vi "GetFltrMode.vi"(8 "错误输入（无错误）":errorcluster) -> (0 "错误输出":errorcluster)   [LabVIEW 2014]
uses:
  X86Dll/ZXUTConfigMgr.dll
panel:
  out "返回值":u16
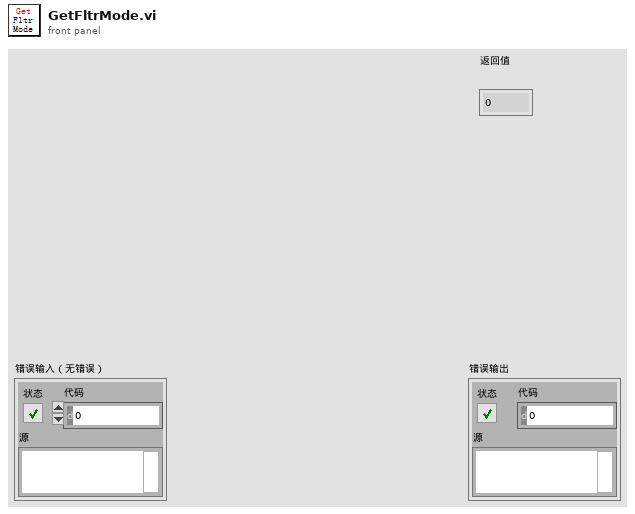
[diagram p1: front panel]
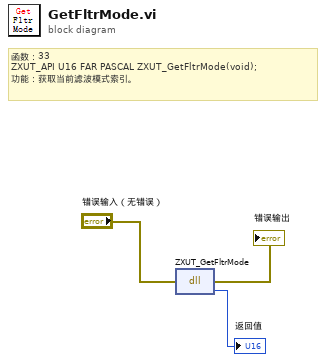
[diagram p0: block diagram]
diagram:
  # "函数：33\nZXUT_API U16\tFAR PASCAL ZXUT_GetFltrMode(void);\n功能：获取当前滤波模式索引。"
  n1 = dll-call lib="D:/Software/Utrasonic on-line monitoring/X86Dll/ZXUTConfigMgr.dll" fn="ZXUT_GetFltrMode"(error in="错误输入（无错误）") -> (error out=→"错误输出":errorcluster, "返回值"=→"返回值":u16)  [unwired: 2 in, 1 out]
